vi "2025.vi"() -> ()   [LabVIEW 2025]
doc: "12312312312312"
panel:
  in  "stop":bool
  out "indicator":i32
  out "Waveform Chart":dbl(graph)
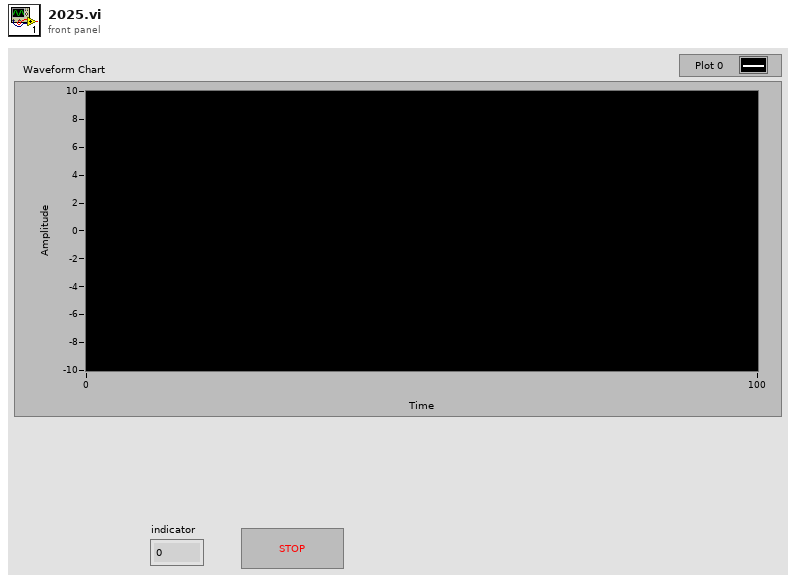
[diagram p1: front panel]
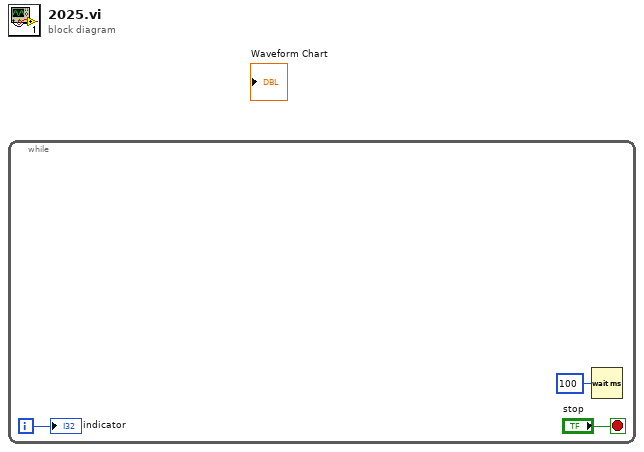
[diagram p0: block diagram]
diagram:
  n1 = while {
    i -> [w1]
    stop <- "stop" stop-if-true
    n2 = Wait (ms)(milliseconds to wait=u32 100) -> ()  [unwired: 1 out]
    "indicator" <- w1
  }
